vi "Close.vi"(8 "error in":errorcluster, 11 "Parallel Mode in":refnum<class "Parallel Mode.lvclass">) -> (0 "error out":errorcluster, 3 "Parallel Mode out":refnum<class "Parallel Mode.lvclass">)   [LabVIEW 2023, in "Parallel Mode.lvclass"]
uses:
  Parallel Mode.lvclass
  Parallel Mode.lvclass/Parallel Mode.ctl
  <vilib>/ADAS Replay HIL/AdasHilServices/AdasHilChannelServices.lvlib
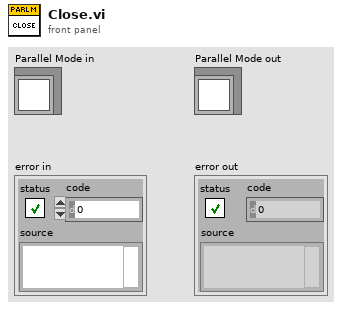
[diagram p1: front panel]
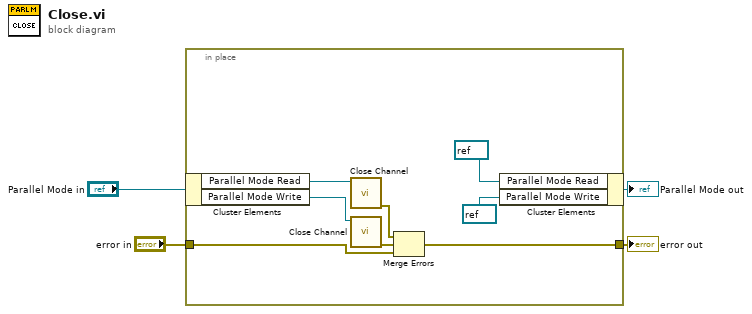
[diagram p0: block diagram]
diagram:
  n1 = in-place {
    in-place-border: "error in" -> [w12]
    in-place-border: [w11] -> w4
    n2 = in-place-cluster #1("Parallel Mode in") -> ("Parallel Mode Read"=w10:refnum<k21>, "Parallel Mode Write"=w9:refnum<k21>)
    n3 = call <vilib>:"Close Channel.vi"("ADAS HIL Channel"=w10) -> ("error out"=w6:errorcluster)  [unwired: 10 in]
    n4 = call <vilib>:"Close Channel.vi"("ADAS HIL Channel"=w9) -> ("error out"=w5:errorcluster)  [unwired: 10 in]
    n5 = Merge Errors(w6, w5, w12) -> (w11:errorcluster)
    n6 = in-place-cluster #1("Parallel Mode Read"=refnum<k21> refnum, "Parallel Mode Write"=refnum<k21> refnum) -> (→"Parallel Mode out":refnum<class "Parallel Mode.lvclass">)
  }
  "error out" <- w4
